vi "DBL Trim NaN.vi"(11 "DBL In":dbl[](array[numeric]) format="%#_f") -> (3 "DBL Out":dbl[](array[numeric]) format="%#_f")   [LabVIEW 2024]
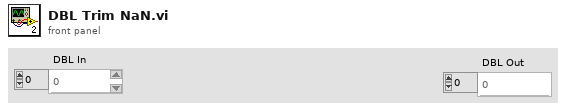
[diagram p1: front panel]
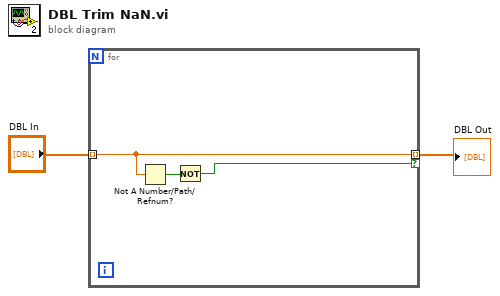
[diagram p0: block diagram]
diagram:
  n1 = for {
    tunnel: "DBL In" -> [w5] mode=indexing
    tunnel: [w5] -> w1 mode=indexing if=w3
    n2 = Not A Number/Path/Refnum?(number/path/refnum=w5) -> (NaN/Path/Refnum?=w4:bool)
    n3 = Not(x=w4) -> (.not. x?=w3:bool)
  }
  "DBL Out" <- w1
